vi "XY Graph Shift Decay to Origin.vi"(8 "error in (no error)":errorcluster, 9 "tolerance factor (1.2)":dbl=1.2, 11 "Decay in":cluster{"t Array":dbl[], "I Array":dbl[]}) -> (0 "error out":errorcluster, 1 "Index of Minimum":i32, 2 "t_0":dbl, 3 "Rotated Decay out":cluster{"t Array":dbl[], "I Array":dbl[]})   [LabVIEW 2021, in "XY Graph Add-Ons.lvlib"]
uses:
  XY Graph Add-Ons.lvlib
  <vilib>/Analysis/NI_AALBase.lvlib
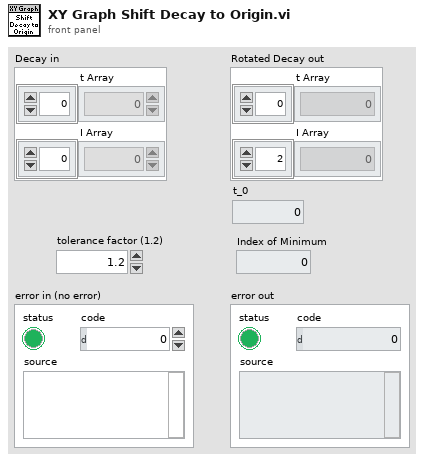
[diagram p1: front panel]
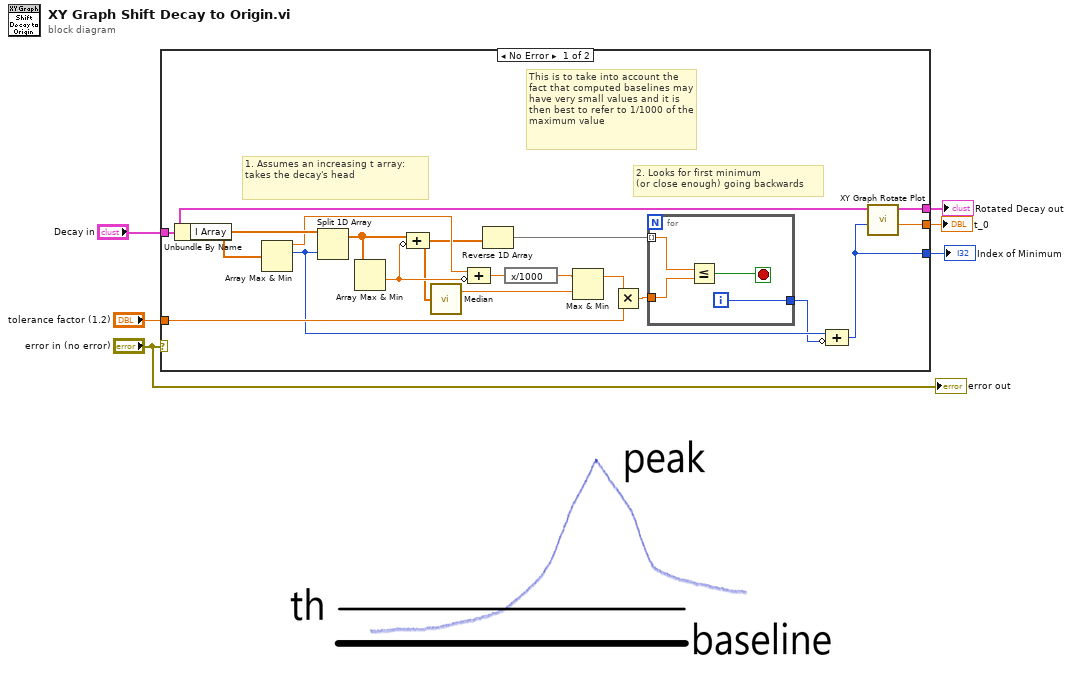
[diagram p0: block diagram]
diagram:
  n1 = case shown="No Error" "error in (no error)" {
    tunnel: "tolerance factor (1.2)" -> [w24 _]
    tunnel: [w14 _] -> w5
    tunnel: [w15 _] -> w4
    tunnel: "Decay in" -> [w16 w29]
    tunnel: [w17 w29] -> w2
    frame No Error {
      # "This is to take into account the fact that computed baselines may have very small values and it is then best to refer to 1/1000 of the maximum value"
      # "2. Looks for first minimum\n(or close enough) going backwards"
      # "1. Assumes an increasing t array:\ntakes the decay's head"
      n2 = Unbundle By Name(w16) -> ("I Array"=w18:dbl[])
      n3 = Array Max & Min(array=w18) -> (max value=w11:dbl, max index (indices)=w20:i32)  [unwired: 2 out]
      n4 = Split 1D Array(array=w18, index=w20) -> (first subarray=w21:dbl[])  [unwired: 1 out]
      n5 = Array Max & Min(array=w21) -> (min value=w9:dbl)  [unwired: 3 out]
      n6 = Compound Arithmetic op=ADD(w21, invert w9) -> (w8:dbl[])
      n7 = call <vilib>:"Median.vi"("X"=w8) -> ("median"=w7:dbl)  [unwired: 1 out]
      n8 = Compound Arithmetic op=ADD(w11, invert w9) -> (w10:dbl)
      n9 = Reverse 1D Array(array=w8) -> (reversed array=w23:dbl[])
      n10 = expression code="x/1000"(w10) -> (w12:dbl)
      n11 = Max & Min(x=w12, y=w7) -> (max(x,y)=w13:dbl)  [unwired: 1 out]
      n12 = Multiply(x=w13, y=w24) -> (x*y=w22:dbl)
      n13 = for {
        tunnel: w23 -> [w27] mode=indexing
        tunnel: w22 -> [w26]
        tunnel: [w28] -> w19
        i -> [w28]
        stop <- w25 stop-if-true
        n14 = Less Or Equal?(x=w27, y=w26) -> (x <= y?=w25:bool)
      }
      n15 = Compound Arithmetic op=ADD(w20, invert w19) -> (w15:i32)
      n16 = call "XY Graph Rotate Plot.vi"("Index of t_0"=w15, "Decay in"=w16) -> ("t_0"=w14:dbl, "Decay out"=w17:cluster{"t Array":dbl[], "I Array":dbl[]})  [unwired: 7 in, 1 out]
    }
    frame Error {
    }
  }
  "Rotated Decay out" <- w2
  "t_0" <- w5
  "Index of Minimum" <- w4
  "error out" <- "error in (no error)"
